vi "Two Servos Example 2.vi"(8 "Error In":errorcluster) -> (0 "Error Out":errorcluster)   [LabVIEW 2014]
doc: "Tested on:\n - Arduino Nano\n\nExample how to rotate two servos."
uses:
  LabVIEW-Universal-Transcriptor-ServoLibrary/ServoDatatype.lvclass
panel:
  in  "Servo2 pin":i32=13
  in  "Servo1 pin":i32=10
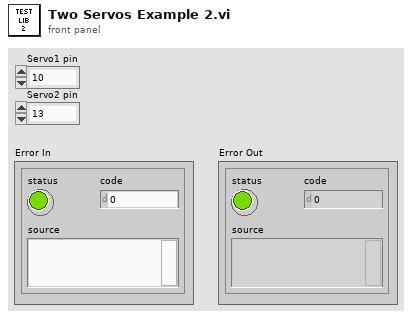
[diagram p1: front panel]
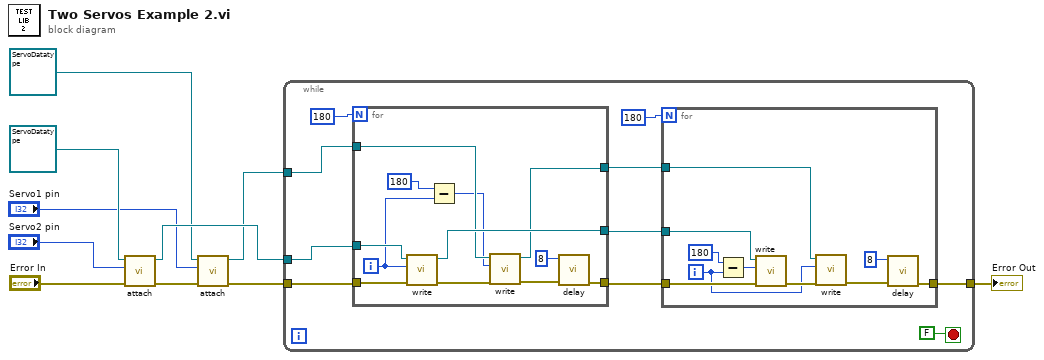
[diagram p0: block diagram]
diagram:
  n1 = call-dynamic "attach.vi"("error in (no error)"="Error In", "pin number"="Servo2 pin", "Servo in"=refnum<class "ServoDatatype.lvclass"> refnum) -> ("error out"=w5:errorcluster, "Servo out"=w7:refnum<class "ServoDatatype.lvclass">)  [unwired: 6 in, 1 out]
  n2 = call-dynamic "attach.vi"("error in (no error)"=w5, "pin number"="Servo1 pin", "Servo in"=refnum<class "ServoDatatype.lvclass"> refnum) -> ("error out"=w4:errorcluster, "Servo out"=w1:refnum<class "ServoDatatype.lvclass">)  [unwired: 6 in, 1 out]
  n3 = while {
    tunnel: w4 -> [w18]
    tunnel: w7 -> [w19]
    tunnel: [w13] -> w6
    tunnel: w1 -> [w12]
    stop <- FALSE stop-if-true
    n4 = for {
      N: 180 -> [_]
      tunnel: w19 -> [w42]
      tunnel: w18 -> [w41]
      tunnel: [w40] -> w16
      tunnel: [w38] -> w14
      tunnel: w12 -> [w35]
      tunnel: [w33] -> w11
      i -> [w32]
      n5 = call-dynamic "write.vi"("error in (no error)"=w41, "value"=w32, "ServoDatatype in"=w42) -> ("error out"=w37:errorcluster, "ServoDatatype out"=w40:refnum<class "ServoDatatype.lvclass">)  [unwired: 7 in]
      n6 = Subtract(x=180, y=w32) -> (x-y=w31:i32)
      n7 = call-dynamic "write.vi"("error in (no error)"=w37, "value"=w31, "ServoDatatype in"=w35) -> ("error out"=w34:errorcluster, "ServoDatatype out"=w33:refnum<class "ServoDatatype.lvclass">)  [unwired: 7 in]
      n8 = call <vilib>:"delay.vi"("Error In"=w34, "time (ms)"=8) -> ("Error Out"=w38:errorcluster)  [unwired: 9 in]
    }
    n9 = for {
      N: 180 -> [_]
      tunnel: w16 -> [w30]
      tunnel: w14 -> [w29]
      tunnel: [w26] -> w13
      tunnel: w11 -> [w24]
      i -> [w21]
      n10 = Subtract(x=180, y=w21) -> (x-y=w22:i32)
      n11 = call-dynamic "write.vi"("error in (no error)"=w29, "value"=w22, "ServoDatatype in"=w30) -> ("error out"=w25:errorcluster)  [unwired: 7 in, 1 out]
      n12 = call-dynamic "write.vi"("error in (no error)"=w25, "value"=w21, "ServoDatatype in"=w24) -> ("error out"=w23:errorcluster)  [unwired: 7 in, 1 out]
      n13 = call <vilib>:"delay.vi"("Error In"=w23, "time (ms)"=8) -> ("Error Out"=w26:errorcluster)  [unwired: 9 in]
    }
  }
  "Error Out" <- w6
